vi "Drive Straight PID.vi"(5 "Angle Offset":dbl, 6 "Iteration":i32, 7 "target distance":dbl, 8 "Period (ms)":i64=10) -> (2 "Right Axis":dbl, 3 "Left Axis":dbl)   [LabVIEW 2019]
uses:
  <vilib>/addons/control/pid/NI_PID_pid.lvlib
  <vilib>/addons/control/pid/pid.llb/PID Output Rate Limiter (DBL).vi
  Odometry/Typedef/Odometry.ctl
  <vilib>/Rock Robotics/WPI/ThirdParty/WPILib Extensions/Geometry/Typedef/Translation2d.ctl
  <vilib>/Rock Robotics/WPI/ThirdParty/WPILib Extensions/Geometry/Typedef/Rotation2d.ctl
  <vilib>/Rock Robotics/WPI/ThirdParty/WPILib Extensions/Geometry/Typedef/Pose2d.ctl
panel:
  in  "Odometry":T1
  in  "output rate":dbl=80.0 format="%.2f"
  in  "Gyro PIDF":cluster{"Kp":dbl, "Ki":dbl, "Kd":dbl, "Kf":dbl}={"Kp"=0.05, "Ki"=0.0, "Kd"=0.0, "Kf"=0.0} {"Kf" format="%.3f"; "Kd" format="%.3f"; "Ki" format="%.3f"; "Kp" format="%.3f"}
  in  "PIDF":cluster{"Kp":dbl, "Ki":dbl, "Kd":dbl, "Kf":dbl}={"Kp"=0.02, "Ki"=0.0, "Kd"=0.045, "Kf"=0.0} {"Kf" format="%.3f"; "Kd" format="%.3f"; "Ki" format="%.3f"; "Kp" format="%.3f"}
  in  "i Zone":dbl=12.0 format="%.2f"
  in  "output range":cluster{"output high":dbl, "output low":dbl}={"output high"=1.0, "output low"=-1.0} {"output low" format="%.2f"; "output high" format="%.2f"}
  out "Waveform Chart 2":cluster{dbl, dbl}(graph)={-50.0, -50.00778875}
  out "Gyro Output":dbl(graph)=0.02713616249999992
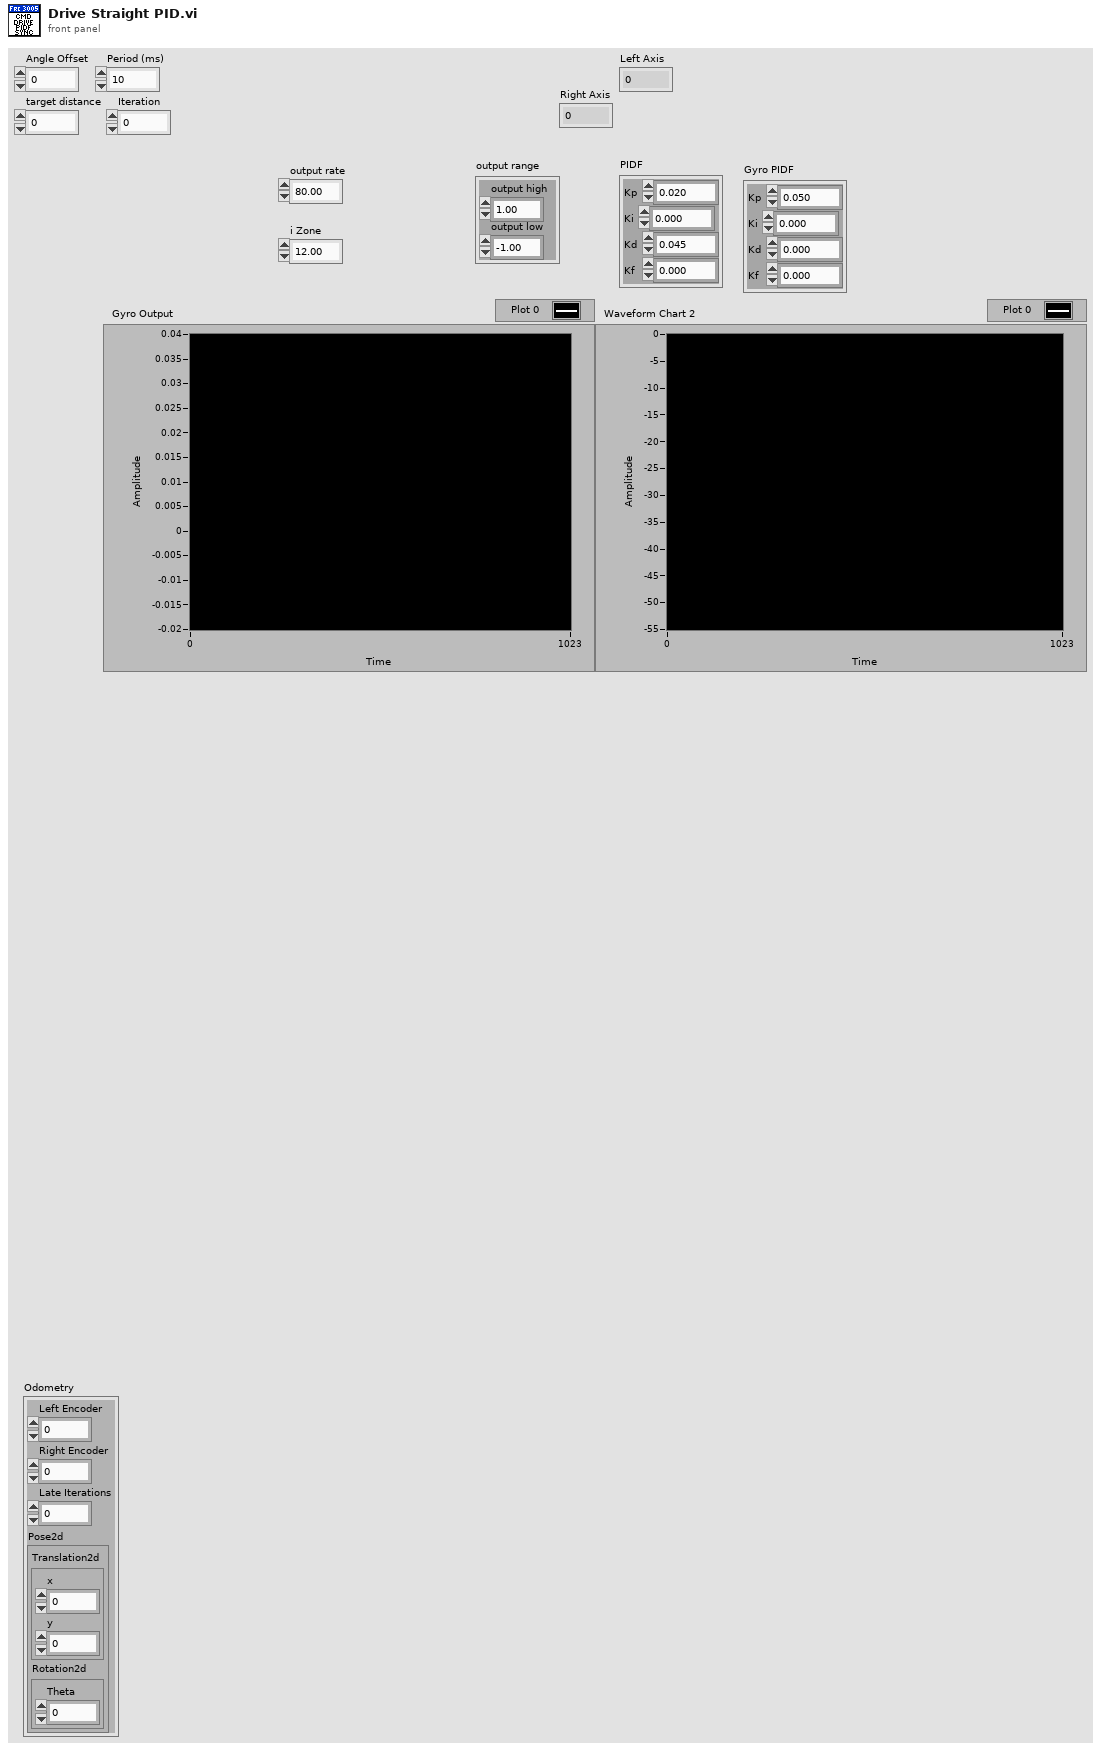
[diagram p1: front panel]
types:
  T1 = typedef "Odometry.ctl" = cluster{"Left Encoder":dbl, "Right Encoder":dbl, "Late Iterations":i16, "Pose2d":T2}
  T2 = typedef "Pose2d.ctl" = cluster{"Translation2d":T3, "Rotation2d":T4}
  T3 = typedef "Translation2d.ctl" = cluster{"x":dbl, "y":dbl}
  T4 = typedef "Rotation2d.ctl" = cluster{"Theta":dbl}
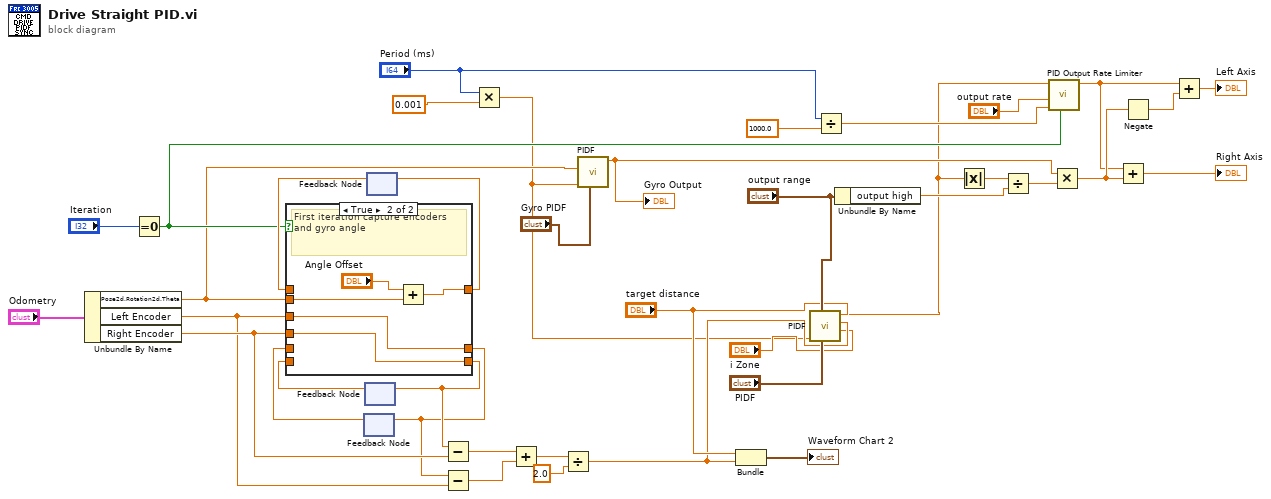
[diagram p0: block diagram]
diagram:
  n1 = Unbundle By Name("Odometry") -> ("Pose2d.Rotation2d.Theta"=w11:dbl, "Left Encoder"=w15:dbl, "Right Encoder"=w17:dbl)
  n2 = Equal To 0?(x="Iteration") -> (x = 0?=w25:bool)
  n3 = feedback #1() -> (w19:dbl)  [unwired: 1 in]
  n4 = feedback #2() -> (w20:dbl)  [unwired: 1 in]
  n5 = feedback #3() -> (w26:dbl)  [unwired: 1 in]
  n6 = case shown="True" w25 {
    tunnel: [w42 w46] -> w27
    tunnel: w26 -> [w42 _]
    tunnel: w11 -> [_ w45]
    tunnel: w15 -> [_ w43]
    tunnel: w17 -> [_ w44]
    tunnel: [w41 w44] -> w18
    tunnel: [w40 w43] -> w16
    tunnel: w20 -> [w41 _]
    tunnel: w19 -> [w40 _]
    frame False {
    }
    frame True {
      # "First iteration capture encoders and gyro angle"
      n7 = Add(x="Angle Offset", y=w45) -> (x+y=w46:dbl)
    }
  }
  n8 = feedback-in #1(w16) -> ()
  n9 = feedback-in #2(w18) -> ()
  n10 = feedback-in #3(w27) -> ()
  n11 = Subtract(x=w18, y=w17) -> (x-y=w14:dbl)
  n12 = Subtract(x=w16, y=w15) -> (x-y=w13:dbl)
  n13 = Multiply(x="Period (ms)", y=0.001) -> (x*y=w1:dbl)
  n14 = Add(x=w14, y=w13) -> (x+y=w39:dbl)
  n15 = Divide(x=w39, y=2.0) -> (x/y=w6:dbl)
  n16 = call <vilib>:"PIDF.vi"("PIDF gains"="Gyro PIDF", "dt (s)"=w1, "process variable"=w11) -> ("output"=w10:dbl)  [unwired: 6 in, 2 out]
  "Gyro Output" <- w10
  n17 = Bundle("target distance"="target distance", w6) -> (→"Waveform Chart 2":cluster{"target distance":dbl, dbl})  [unwired: 1 in]
  n18 = call <vilib>:"PIDF.vi"("PIDF gains"="PIDF", "output range"="output range", "dt (s)"=w1, "i Zone"="i Zone", "process variable"=w6, "setpoint"="target distance") -> ("output"=w4:dbl)  [unwired: 3 in, 2 out]
  n19 = Divide(x="Period (ms)", y=1000.0) -> (x/y=w35:dbl)
  n20 = Unbundle By Name("output range") -> ("output high"=w31:dbl)
  n21 = Absolute Value(x=w4) -> (abs(x)=w22:dbl)
  n22 = Divide(x=w22, y=w31) -> (x/y=w30:dbl)
  n23 = call-poly <vilib>:"PID Output Rate Limiter.vi"("reinitialize? (F)"=w25, "dt (s)"=w35, "output rate (EGU/min)"="output rate", "input (controller output)"=w4) -> ("output"=w28:dbl)  [unwired: 4 in, 1 out]
  n24 = Multiply(x=w10, y=w30) -> (x*y=w32:dbl)
  n25 = Add(x=w28, y=w32) -> (x+y=→"Right Axis":dbl)
  n26 = Negate(x=w32) -> (-x=w33:dbl)
  n27 = Add(x=w28, y=w33) -> (x+y=→"Left Axis":dbl)
